vi "Receiver.vi"() -> ()   [LabVIEW 2020]
uses:
  vi.lib/MakerHub/PS4-Controller/Private/Type Defs/Indicators/Controller.ctl
  vi.lib/MakerHub/PS4-Controller/Private/Type Defs/Indicators/Square.ctl
  vi.lib/MakerHub/PS4-Controller/Private/Type Defs/Indicators/X.ctl
  vi.lib/MakerHub/PS4-Controller/Private/Type Defs/Indicators/Circle.ctl
  vi.lib/MakerHub/PS4-Controller/Private/Type Defs/Indicators/Triangle.ctl
  vi.lib/MakerHub/PS4-Controller/Private/Type Defs/Indicators/L1.ctl
  vi.lib/MakerHub/PS4-Controller/Private/Type Defs/Indicators/R1.ctl
  vi.lib/MakerHub/PS4-Controller/Private/Type Defs/Indicators/Share.ctl
  vi.lib/MakerHub/PS4-Controller/Private/Type Defs/Indicators/Options.ctl
  vi.lib/MakerHub/PS4-Controller/Private/Type Defs/Indicators/PS.ctl
  vi.lib/MakerHub/PS4-Controller/Private/Type Defs/Indicators/Pad_Button.ctl
  vi.lib/MakerHub/PS4-Controller/Private/Type Defs/Indicators/Dpad.ctl
  vi.lib/MakerHub/PS4-Controller/Private/Type Defs/Indicators/Slider.ctl
  <vilib>/ReMiSYS Technology/RemoteToolkit/Receiver/Receiver.lvclass
  vi.lib/MakerHub/PS4-Controller/LMH-PS4.lvlib
panel:
  out "PS4 Controller":T1={"Square Button"=FALSE, "X Button"=FALSE, "Circle Button"=FALSE, "Triangle Button"=FALSE, "L1"=FALSE, "R1"=FALSE, "Share Button"=FALSE, "Options Button"=FALSE, "PS Button"=FALSE, "Pad Button"=FALSE, "D-Pad"=5, "L2"=0, "R2"=0, "Thumbstick_Left"={[], []}, "Thumbstick_Right"={[], []}} {"R2" scale=-32768.0..32767.0; "L2" scale=-32768.0..32767.0}
  out "Error Out":errorcluster
  out "Received?":bool
  in  "Stop":bool
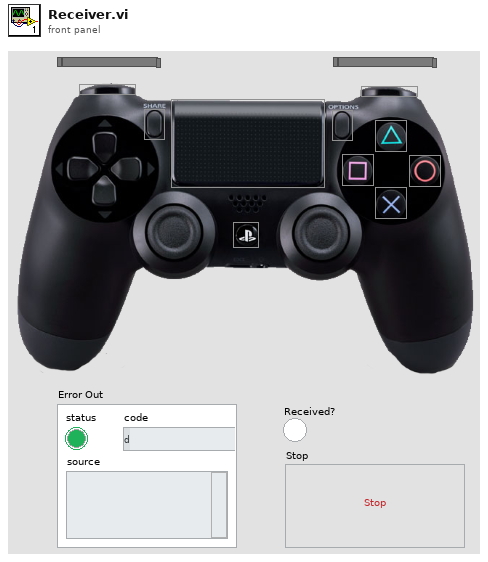
[diagram p1: front panel]
types:
  T1 = typedef "LMH-PS4.lvlib/Controller.ctl" = cluster{"Square Button":T2, "X Button":T3, "Circle Button":T4, "Triangle Button":T5, "L1":T6, "R1":T7, "Share Button":T8, "Options Button":T9, "PS Button":T10, "Pad Button":T11, "D-Pad":T12, "L2":T13, "R2":T13, "Thumbstick_Left":cluster{i32[], i32[]}, "Thumbstick_Right":cluster{i32[], i32[]}}
  T2 = typedef "LMH-PS4.lvlib/Square.ctl" = bool
  T3 = typedef "LMH-PS4.lvlib/X.ctl" = bool
  T4 = typedef "LMH-PS4.lvlib/Circle.ctl" = bool
  T5 = typedef "LMH-PS4.lvlib/Triangle.ctl" = bool
  T6 = typedef "LMH-PS4.lvlib/L1.ctl" = bool
  T7 = typedef "LMH-PS4.lvlib/R1.ctl" = bool
  T8 = typedef "LMH-PS4.lvlib/Share.ctl" = bool
  T9 = typedef "LMH-PS4.lvlib/Options.ctl" = bool
  T10 = typedef "LMH-PS4.lvlib/PS.ctl" = bool
  T11 = typedef "LMH-PS4.lvlib/Pad_Button.ctl" = bool
  T12 = typedef "LMH-PS4.lvlib/Dpad.ctl" = u16
  T13 = typedef "LMH-PS4.lvlib/Slider.ctl" = i32
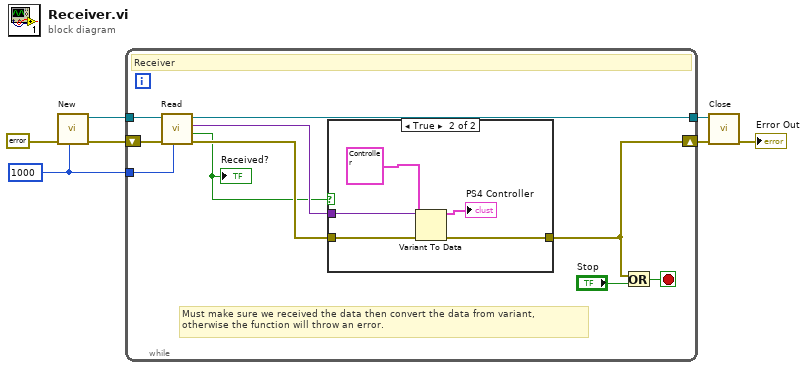
[diagram p0: block diagram]
diagram:
  w3 = 1000 ("Timeout ms (25000)")
  n1 = call <vilib>:"New.vi"("Timeout ms (25000)"=w3, "Error In"=errorcluster {"status"=FALSE, "code"=0, "source"=""}) -> ("Error Out"=w7:errorcluster, "Receiver Ref."=w6:refnum<class "Receiver.lvclass">)  [unwired: 8 in]
  n2 = while {
    shift-right: [w9] -> w5
    shift-left: w7 -> [w17]
    tunnel: w6 -> [w16]
    tunnel: [w15] -> w4
    tunnel: w3 -> [w14]
    stop <- w12 stop-if-true
    # "Must make sure we received the data then convert the data from variant,\notherwise the function will throw an error."
    # "Receiver"
    n3 = call <vilib>:"Read.vi"("Timeout ms (1000)"=w14, "Error In"=w17, "Receiver Ref."=w16) -> ("Error Out"=w11:errorcluster, "Received?"=w8:bool, "Value"=w10:variant, "Receiver Ref."=w15:refnum<class "Receiver.lvclass">)  [unwired: 5 in]
    "Received?" <- w8
    n4 = case shown="True" w8 {
      tunnel: w11 -> [w18 w23]
      tunnel: w10 -> [_ w22]
      tunnel: [w18 w21] -> w9
      frame False {
      }
      frame True {
        n5 = Variant To Data(error in=w23, type=T1 {"Square Button"=FALSE, "X Button"=FALSE, "Circle Button"=FALSE, "Triangle Button"=FALSE, "L1"=FALSE, "R1"=FALSE, "Share Button"=FALSE, "Options Button"=FALSE, "PS Button"=FALSE, "Pad Button"=FALSE, "D-Pad"=0, "L2"=-32768, "R2"=-32768, "Thumbstick_Left"={[0, 0], [0, 0]}, "Thumbstick_Right"={[0, 0], [0, 0]}} ("PS4 Controller"), Variant=w22) -> (data=→"PS4 Controller":T1, error out=w21:errorcluster)
      }
    }
    n6 = Or(x=w9, y="Stop") -> (x .or. y?=w12:bool)
  }
  n7 = call <vilib>:"Close.vi"("Error In"=w5, "Receiver Ref."=w4) -> ("Error Out"=→"Error Out":errorcluster)  [unwired: 9 in]
